vi "GOOP_UMLEditor_CallMain.vi"(0 "AppRef":refnum<vi>, 1 "Enum":T1, 2 "Project":string, 3 "Class/VI-Path":path, 4 "Target":string, 5 "error in (no error)":errorcluster) -> (19 "error out":errorcluster)   [LabVIEW 2014]
uses:
  <resource>/Framework/Providers/Open_GDS/SubVIs/GOOP_UMLEditor_CallMainAction.ctl
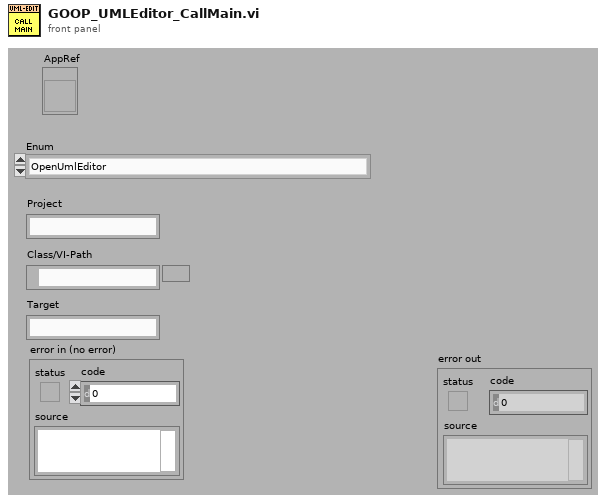
[diagram p1: front panel]
types:
  T1 = typedef "GOOP_UMLEditor_CallMainAction.ctl" = enum16{"OpenUmlEditor", "ReverseEngineering:WholeProject", "ReverseEngineering:OneClass", "ReverseEngineering:OneVI", "ShowInStateDiagram:OneVI", "OpenUMLFile"}
  T2 = enum32{"Bad", "Idle", "Run top level", "Running"}
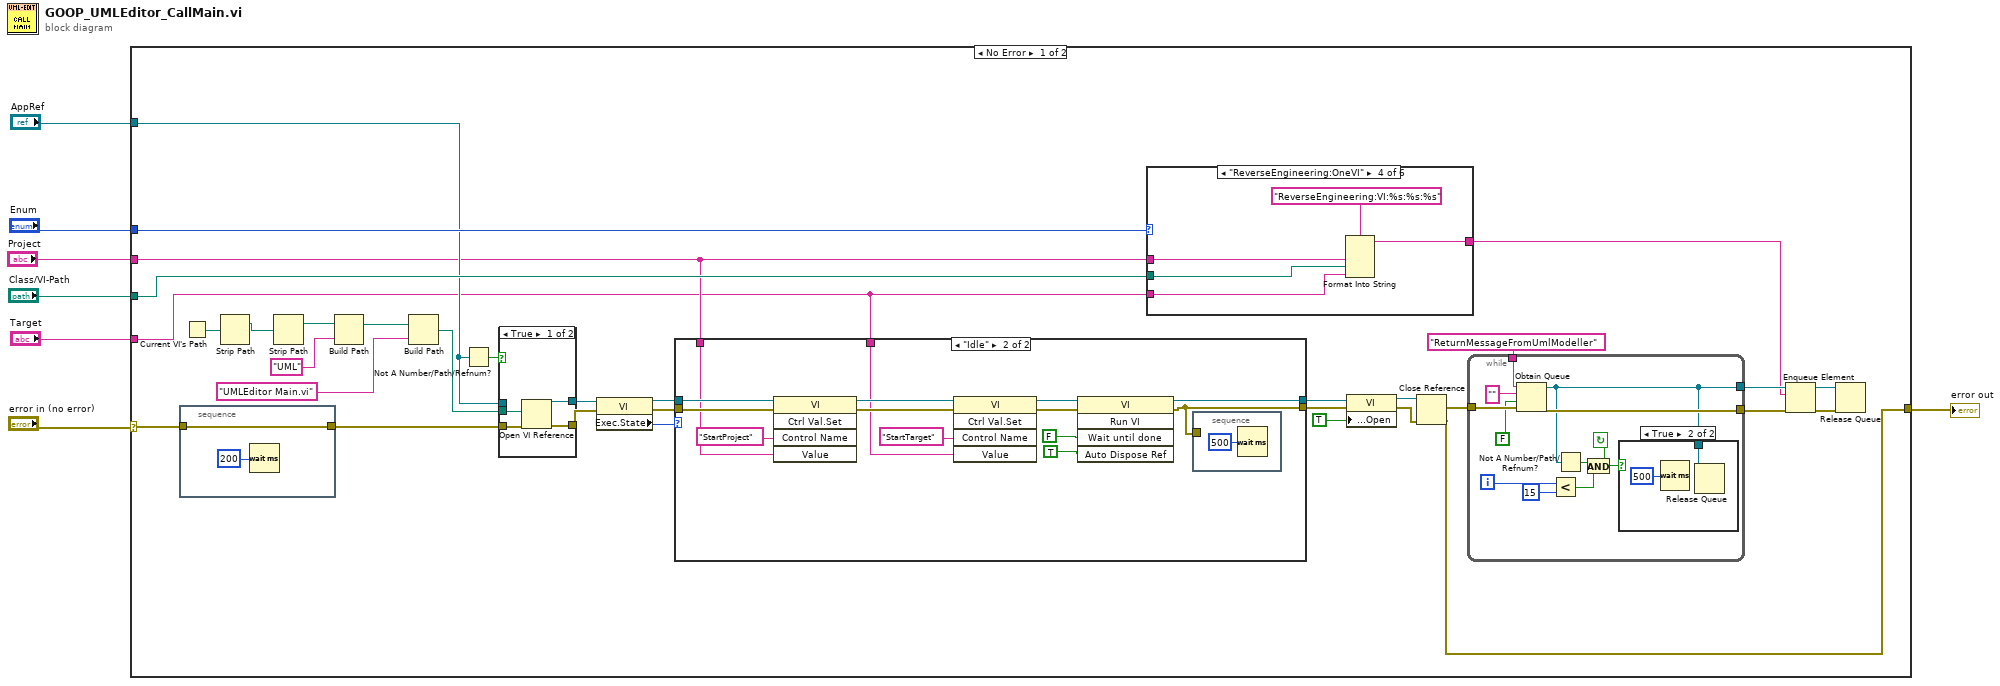
[diagram p0: block diagram]
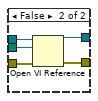
[diagram p2: hidden frame]
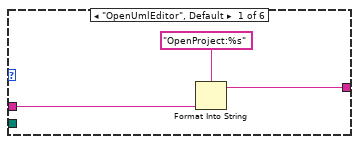
[diagram p4: hidden frame]
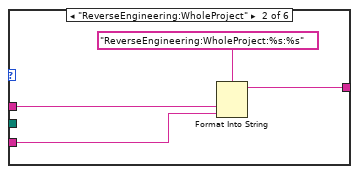
[diagram p5: hidden frame]
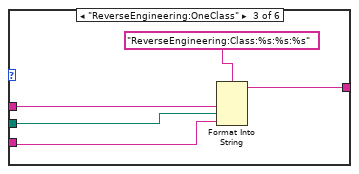
[diagram p6: hidden frame]
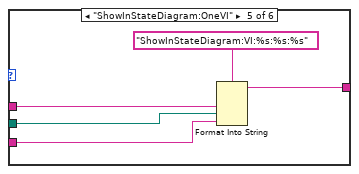
[diagram p7: hidden frame]
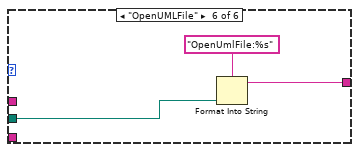
[diagram p8: hidden frame]
diagram:
  n1 = case shown="No Error" "error in (no error)" {
    selector: "error in (no error)" -> [w16 w106]
    tunnel: "Enum" -> [w24 _]
    tunnel: [w12 w106] -> w5
    tunnel: "Project" -> [w9 _]
    tunnel: "Class/VI-Path" -> [w17 _]
    tunnel: "AppRef" -> [w10 _]
    tunnel: "Target" -> [w8 _]
    frame No Error {
      n2 = stacked-sequence {
        tunnel: [w50] -> w15
        tunnel: w16 -> [w50]
        frame #0 {
          n3 = Wait (ms)(milliseconds to wait=u32 200) -> ()  [unwired: 1 out]
        }
      }
      n4 = Current VI's Path() -> (path=w39:path)
      n5 = Strip Path(path=w39) -> (stripped path=w38:path)  [unwired: 1 out]
      n6 = Strip Path(path=w38) -> (stripped path=w37:path)  [unwired: 1 out]
      n7 = Build Path(base path=w37, name or relative path="UML") -> (appended path=w35:path)
      n8 = Build Path(base path=w35, name or relative path="UMLEditor Main.vi") -> (appended path=w33:path)
      n9 = Not A Number/Path/Refnum?(number/path/refnum=w10) -> (NaN/Path/Refnum?=w11:bool)
      n10 = case shown="True" w11 {
        tunnel: w33 -> [w43 w48]
        tunnel: [w42 w47] -> w32
        tunnel: [w41 w46] -> w31
        tunnel: w15 -> [w40 w45]
        tunnel: w10 -> [_ w44]
        frame True {
          n11 = Open VI Reference(vi path=w43, error in (no error)=w40) -> (vi reference=w42:refnum<vi>, error out=w41:errorcluster)  [unwired: 4 in]
        }
        frame False {
          n12 = Open VI Reference(application reference (local)=w44, vi path=w48, error in (no error)=w45) -> (vi reference=w47:refnum<vi>, error out=w46:errorcluster)  [unwired: 3 in]
        }
      }
      n13 = property class="VI"(reference=w32, error in=w31) -> (reference out=w29:refnum<vi>, error out=w28:errorcluster, "Exec.State"=w30:T2)
      n14 = case shown="\"Idle\"" w30 {
        tunnel: w29 -> [w90 w100]
        tunnel: w28 -> [w89 w99]
        tunnel: [w90 w103] -> w27
        tunnel: [w89 w101] -> w26
        tunnel: w9 -> [_ w97]
        tunnel: w8 -> [_ w91]
        frame "Bad", Default {
        }
        frame "Idle" {
          n15 = invoke class="VI" method="Ctrl Val.Set"(reference=w100, error in=w99, "Control Name"="StartProject", "Value"=w97) -> (reference out=w96:refnum<vi>, error out=w95:errorcluster)  [unwired: 1 in, 3 out]
          n16 = invoke class="VI" method="Ctrl Val.Set"(reference=w96, error in=w95, "Control Name"="StartTarget", "Value"=w91) -> (reference out=w92:refnum<vi>, error out=w93:errorcluster)  [unwired: 1 in, 3 out]
          n17 = invoke class="VI" method="Run VI"(reference=w92, error in=w93, "Wait until done"=FALSE ("Wait Until Done"), "Auto Dispose Ref"=TRUE ("Front Panel Window:Open")) -> (reference out=w103:refnum<vi>, error out=w101:errorcluster)  [unwired: 1 in, 3 out]
          n18 = stacked-sequence {
            tunnel: w101 -> [_]
            frame #0 {
              n19 = Wait (ms)(milliseconds to wait=u32 500) -> ()  [unwired: 1 out]
            }
          }
        }
      }
      n20 = case shown="\"ReverseEngineering:OneVI\"" w24 {
        tunnel: w9 -> [w65 w69 w74 w79 w84 _]
        tunnel: [w64 w68 w73 w78 w83 w87] -> w18
        tunnel: w17 -> [_ _ w72 w77 w82 w86]
        tunnel: w8 -> [_ w67 w71 w76 w81 _]
        frame "OpenUmlEditor", Default {
          n21 = Format Into String(format string="OpenProject:%s", w65) -> (resulting string=w64:string)  [unwired: 2 in, 1 out]
        }
        frame "ReverseEngineering:WholeProject" {
          n22 = Format Into String(format string="ReverseEngineering:WholeProject:%s:%s", w69, w67) -> (resulting string=w68:string)  [unwired: 2 in, 1 out]
        }
        frame "ReverseEngineering:OneClass" {
          n23 = Format Into String(format string="ReverseEngineering:Class:%s:%s:%s", w74, w72, w71) -> (resulting string=w73:string)  [unwired: 2 in, 1 out]
        }
        frame "ReverseEngineering:OneVI" {
          n24 = Format Into String(format string="ReverseEngineering:VI:%s:%s:%s", w79, w77, w76) -> (resulting string=w78:string)  [unwired: 2 in, 1 out]
        }
        frame "ShowInStateDiagram:OneVI" {
          n25 = Format Into String(format string="ShowInStateDiagram:VI:%s:%s:%s", w84, w82, w81) -> (resulting string=w83:string)  [unwired: 2 in, 1 out]
        }
        frame "OpenUMLFile" {
          n26 = Format Into String(format string="OpenUmlFile:%s", w86) -> (resulting string=w87:string)  [unwired: 2 in, 1 out]
        }
      }
      n27 = property class="VI"(reference=w27, error in=w26, "Front Panel.Open"=TRUE ("Front Panel Window:Open")) -> (reference out=w14:refnum<vi>, error out=w13:errorcluster)
      n28 = Close Reference(reference=w14, error in (no error)=w13) -> (error out=w12:errorcluster)
      n29 = while {
        tunnel: "ReturnMessageFromUmlModeller" ("name (unnamed)") -> [w61]
        tunnel: [w51] -> w22
        tunnel: [w52] -> w21
        tunnel: w12 -> [w60]
        i -> [w58]
        stop <- w55 continue-if-true
        n30 = Obtain Queue(name (unnamed)=w61, element data type="", create if not found? (T)=FALSE, error in (no error)=w60) -> (queue out=w51:refnum<queue>, error out=w52:errorcluster)  [unwired: 1 in, 1 out]
        n31 = Less?(x=w58, y=15) -> (x < y?=w56:bool)
        n32 = Not A Number/Path/Refnum?(number/path/refnum=w51) -> (NaN/Path/Refnum?=w57:bool)
        n33 = Compound Arithmetic op=AND(w57, w56) -> (w55:bool)
        n34 = case shown="True" w55 {
          tunnel: w51 -> [_ w62]
          frame False {
          }
          frame True {
            n35 = Wait (ms)(milliseconds to wait=u32 500) -> ()  [unwired: 1 out]
            n36 = Release Queue(queue=w62) -> ()  [unwired: 2 in, 3 out]
          }
        }
      }
      n37 = Enqueue Element(queue=w22, element=w18, error in (no error)=w21) -> (queue out=w20:refnum<queue>, error out=w19:errorcluster)  [unwired: 1 in, 1 out]
      n38 = Release Queue(queue=w20, error in (no error)=w19) -> ()  [unwired: 1 in, 3 out]
    }
    frame Error {
    }
  }
  "error out" <- w5
